vi "Autonomous Independent.vi"() -> ()   [LabVIEW 2013]
doc: "This VI is called when autonomous begins, and will automatically be terminated when autonomous ends. You can carry out timed or sensor driven robot movement independently without needing to return to the caller."
uses:
  Robot Global Data.vi
  OneBall.ctl
  DoubleSolenoidControl.ctl
  RollerStates.ctl
  ShooterAction.ctl
panel:
  out "Error out":errorcluster
  in  "Error in":errorcluster
  # "Be sure to right-click and choose Data Operations>>Make Current Value default if you want to save the array values with the VI"
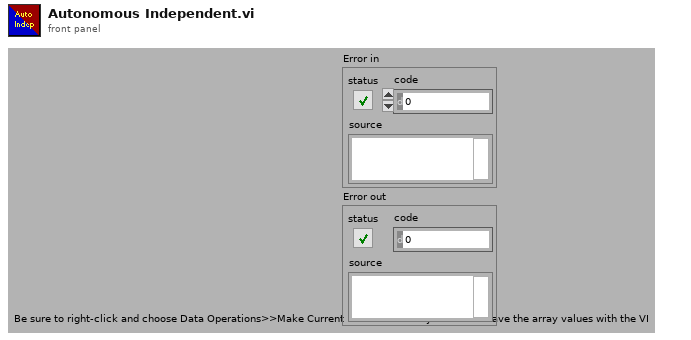
[diagram p1: front panel]
types:
  T1 = typedef "OneBall.ctl" = enum16{"Init", "Drive", "Shoot", "CheckGoal", "Stop"}
  T2 = typedef "WPI_JoystickDevRef.ctl" = cluster{"Device":T3}
  T3 = typedef "WPI_JoystickDeviceEnum.ctl" = enum16{"USB 1", "USB 2", "USB 3", "USB 4", "Kinect 1", "Kinect 2"}
  T4 = cluster{"axis 1 (x)":dbl, "axis 2 (y)":dbl, "axis 3 (throttle)":dbl, "axis 4":dbl, "axis 5":dbl, "axis 6":dbl}
  T5 = typedef "DoubleSolenoidControl.ctl" = enum16{"Init", "Out", "In", "Middle"}
  T6 = typedef "RollerStates.ctl" = enum16{"Init", "Off", "Forward", "Reverse"}
  T7 = typedef "ShooterAction.ctl" = enum16{"Init", "Shoot"}
  T8 = typedef "WPI_RelayDevRef.ctl" = cluster{"DevStatus":errorcluster, "Relay Channel":T9, "Digital Module":T10, "Relay Direction":T11}
  T9 = typedef "FPGA_DIORelayChannel.ctl" = enum8{"Relay 1", "Relay 2", "Relay 3", "Relay 4", "Relay 5", "Relay 6", "Relay 7", "Relay 8", "Invalid"}
  T10 = typedef "FPGA_TypedefDigitalModule.ctl" = enum16{"Digital Module 1", "Digital Module 2"}
  T11 = typedef "WPI_RelayDirection.ctl" = enum16{"Both directions", "Forward only", "Reverse only"}
  T12 = typedef "WPI_SolenoidDevRef.ctl" = cluster{"DevStatus":errorcluster, "Solenoid Module":T13, "Forward Solenoid Channel":T14, "Reverse Solenoid Channel":T14}
  T13 = typedef "FPGA_TypedefSolenoidModule.ctl" = enum16{"Solenoid Module 1", "Solenoid Module 2"}
  T14 = typedef "WPI_SolenoidChannel.ctl" = enum8{"Solenoid 1", "Solenoid 2", "Solenoid 3", "Solenoid 4", "Solenoid 5", "Solenoid 6", "Solenoid 7", "Solenoid 8", "Invalid"}
  T15 = typedef "WPI_MotorControlDeviceRef.ctl" = cluster{"DeviceStatus":errorcluster, "Type":enum16{"PWM", "CAN"}, "PWM":cluster{"Digital Module":T10, "PWM Channel":T16, "DeadBand":T17}, "CAN":cluster{"Device Number":u8, "Control Mode":T18, "Semaphore":T19, "Max Vout":dbl}, "Invert":bool, "TransformRef":T20, "InvTransformRef":T20}
  T16 = typedef "FPGA_DIOPWMChannel.ctl" = enum8{"PWM 1", "PWM 2", "PWM 3", "PWM 4", "PWM 5", "PWM 6", "PWM 7", "PWM 8", "PWM 9", "PWM 10", "Invalid"}
  T17 = typedef "WPI_PWMDeadband.ctl" = cluster{"Name":string, "maxPositivePwm":i32, "minPositivePwm":i32, "centerPwm":i32, "maxNegativePwm":i32, "minNegativePwm":i32, "angularRange":u16}
  T18 = typedef "WPI_CANJaguar_ControlMode.ctl" = enum8{"Percent VBus", "Current", "Speed", "Position", "Voltage"}
  T19 = typedef "Semaphore RefNum" = refnum<k1>
  T20 = typedef "WPI_PWMTransform_ConPane.ctl" = refnum<vi>
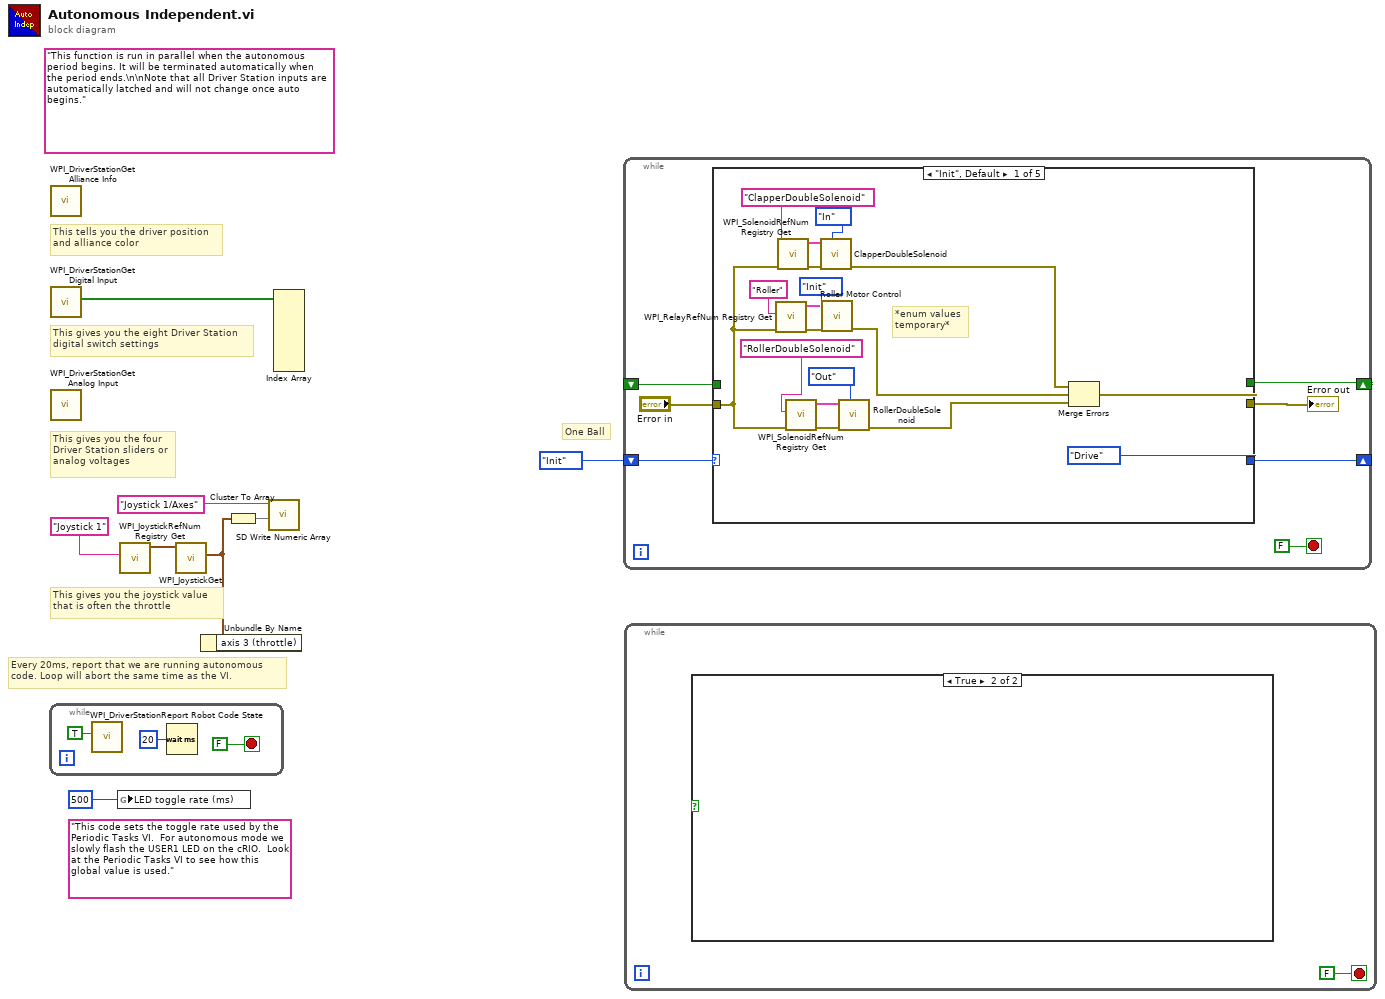
[diagram p0: block diagram]
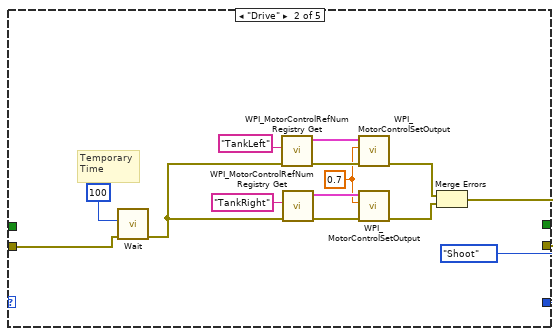
[diagram p3: hidden frame]
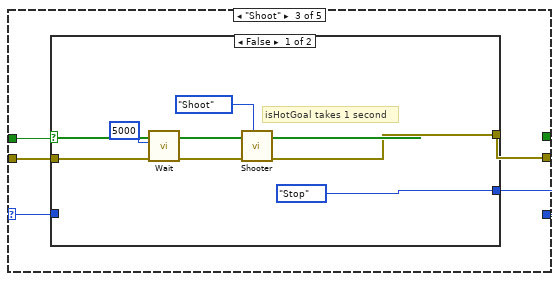
[diagram p4: hidden frame]
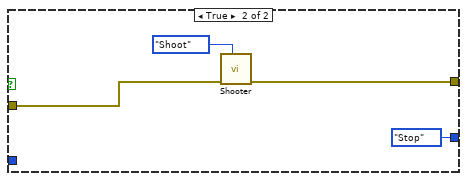
[diagram p5: hidden frame]
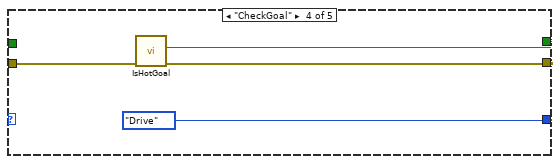
[diagram p6: hidden frame]
diagram:
  (unwired) "This code sets the toggle rate used by the Periodic Tasks VI.  For autonomous mode we slowly flash the USER1 LED on the cRIO.  Look at the Periodic Tasks VI to see how this global value is used."
  (unwired) "This function is run in parallel when the autonomous period begins. It will be terminated automatically when the period ends.\n\nNote that all Driver Station inputs are automatically latched and will not change once auto begins."
  # "One Ball"
  # "Every 20ms, report that we are running autonomous\ncode. Loop will abort the same time as the VI."
  # "This gives you the joystick value\nthat is often the throttle"
  # "This tells you the driver position\nand alliance color"
  # "This gives you the eight Driver Station\ndigital switch settings"
  # "This gives you the four\nDriver Station sliders or\nanalog voltages"
  n1 = while {
    stop <- FALSE stop-if-true
    n2 = call <vilib>:"WPI_DriverStationReport Robot Code State.vi"("Autonomous"=TRUE) -> ()  [unwired: 10 in, 1 out]
    n3 = Wait (ms)(milliseconds to wait=u32 20) -> ()  [unwired: 1 out]
  }
  n4 = call <vilib>:"WPI_DriverStationGet Alliance Info.vi"() -> ()  [unwired: 12 out]
  n5 = call <vilib>:"WPI_DriverStationGet Digital Input.vi"() -> ("Driver Station Digital Input (1-8)"=w8:bool[])  [unwired: 11 out]
  n6 = call <vilib>:"WPI_DriverStationGet Analog Input.vi"() -> ()  [unwired: 12 out]
  n7 = global write "Robot Global Data.vi" "LED toggle rate (ms)"(u32 500 ("LED ms toggle rate")) -> ()
  n8 = call <vilib>:"WPI_JoystickRefNum Registry Get.vi"("refnum name"="Joystick 1") -> ("JoystickDevRef"=w6:T2)  [unwired: 1 in, 9 out]
  n9 = call <vilib>:"WPI_JoystickGet.vi"("JoystickDevRef"=w6) -> ("Axes"=w2:T4)  [unwired: 1 in, 5 out]
  n10 = Unbundle By Name(w2) -> ()  [unwired: 1 out]
  n11 = Cluster To Array(cluster=w2) -> (array=w4:dbl[])
  n12 = call <vilib>:"SD Write Numeric Array.vi"("Numeric Array"=w4, "Name"="Joystick 1/Axes") -> ()  [unwired: 8 in, 2 out]
  n13 = Index Array(array=w8) -> ()  [unwired: 8 in, 8 out]
  n14 = while {
    shift-right: [w15] -> _
    shift-left: OneBall."Init" -> [w14]
    shift-right: [w13] -> _
    shift-left: _ -> [w12]
    stop <- FALSE stop-if-true
    n15 = case shown="\"Init\", Default" w14 {
      selector: w14 -> [_ _ w54 _ _]
      tunnel: [w32 w40 w51 w68 w70] -> w18
      tunnel: "Error in" -> [w20 w41 w52 w69 w70]
      tunnel: [OneBall."Drive" OneBall."Shoot" w55 OneBall."Drive" _] -> w15
      tunnel: [_ _ _ w66 _] -> w13
      tunnel: w12 -> [_ _ w53 _ _]
      frame "Init", Default {
        # "*enum values\ntemporary*"
        n16 = call <vilib>:"WPI_RelayRefNum Registry Get.vi"("error in (no error)"=w20, "refnum name"="Roller") -> ("error out"=w29:errorcluster, "RelayDevRef"=w33:T8)  [unwired: 8 in]
        n17 = call <vilib>:"WPI_SolenoidRefNum Registry Get.vi"("error in (no error)"=w20, "refnum name"="ClapperDoubleSolenoid") -> ("error out"=w28:errorcluster, "SolenoidDevRef"=w35:T12)  [unwired: 8 in]
        n18 = call <vilib>:"WPI_SolenoidRefNum Registry Get.vi"("error in (no error)"=w20, "refnum name"="RollerDoubleSolenoid") -> ("error out"=w23:errorcluster, "SolenoidDevRef"=w24:T12)  [unwired: 8 in]
        n19 = call "ClapperDoubleSolenoid.vi"("State"=DoubleSolenoidControl."In", "Error in"=w28, "SolenoidDevRef"=w35) -> ("Error out"=w31:errorcluster)  [unwired: 8 in]
        n20 = call "Roller Motor Control.vi"("Error in"=w29, "RollerState"=RollerStates."Init", "RelayDevRef"=w33) -> ("Error out"=w30:errorcluster)  [unwired: 8 in]
        n21 = call "RollerDoubleSolenoid.vi"("State"=DoubleSolenoidControl."Out", "Error in"=w23, "SolenoidDevRef"=w24) -> ("Error out"=w22:errorcluster)  [unwired: 8 in]
        n22 = Merge Errors(w31, w30, w22) -> (w32:errorcluster)
      }
      frame "Drive" {
        w45 = 0.7 ("Output")
        # "Temporary\nTime"
        n23 = call "Wait.vi"("error in"=w41, "milliseconds to wait"=u32 100) -> ("error out"=w50:errorcluster)  [unwired: 9 in]
        n24 = call <vilib>:"WPI_MotorControlRefNum Registry Get.vi"("error in (no error)"=w50, "refnum name"="TankLeft") -> ("error out"=w48:errorcluster, "MotorControlDevRef"=w46:T15)  [unwired: 8 in]
        n25 = call <vilib>:"WPI_MotorControlRefNum Registry Get.vi"("error in (no error)"=w50, "refnum name"="TankRight") -> ("error out"=w49:errorcluster, "MotorControlDevRef"=w47:T15)  [unwired: 8 in]
        n26 = call <vilib>:"WPI_MotorControlSetOutput.vi"("error in (no error)"=w48, "Output"=w45, "MotorControlDevRef"=w46) -> ("error out"=w39:errorcluster)  [unwired: 6 in, 2 out]
        n27 = call <vilib>:"WPI_MotorControlSetOutput.vi"("error in (no error)"=w49, "Output"=w45, "MotorControlDevRef"=w47) -> ("error out"=w38:errorcluster)  [unwired: 6 in, 2 out]
        n28 = Merge Errors(w39, w38) -> (w40:errorcluster)
      }
      frame "Shoot" {
        n29 = case shown="False" w53 {
          tunnel: w54 -> [_ _]
          tunnel: [OneBall."Stop" OneBall."Stop"] -> w55
          tunnel: w52 -> [w60 w64]
          tunnel: [w58 w63] -> w51
          frame False {
            # "isHotGoal takes 1 second"
            n30 = call "Wait.vi"("error in"=w60, "milliseconds to wait"=u32 5000) -> ("error out"=w59:errorcluster)  [unwired: 9 in]
            n31 = call "Shooter.vi"("Action"=ShooterAction."Shoot", "error in"=w59) -> ("error out"=w58:errorcluster)  [unwired: 9 in]
          }
          frame True {
            n32 = call "Shooter.vi"("Action"=ShooterAction."Shoot", "error in"=w64) -> ("error out"=w63:errorcluster)  [unwired: 9 in]
          }
        }
      }
      frame "CheckGoal" {
        n33 = call "IsHotGoal.vi"("error in"=w69) -> ("error out"=w68:errorcluster, "Hot/Not"=w66:bool)  [unwired: 9 in]
      }
      frame "Stop" {
      }
    }
    "Error out" <- w18
  }
  n34 = while {
    stop <- FALSE stop-if-true
    n35 = case shown="True" {
      selector: _ -> [_ _]
      frame False {
      }
      frame True {
      }
    }
  }
